vi "SWERVE_DRIVE_SET_SPEED_DEMAND.vi"(8 "Drv Rotation Orentation Dmd":dbl, 9 "Drv Angular Vel Dmd":dbl, 10 "Drv Y Vel Dmd":dbl, 11 "Drv X Vel Dmd":dbl) -> ()   [LabVIEW 2019]
uses:
  SWERVE_DRIVE_GLOBALS.vi
  <vilib>/Rock Robotics/WPI/ThirdParty/JAS_Junk/TrajLib/Trajectory_Library.lvlib
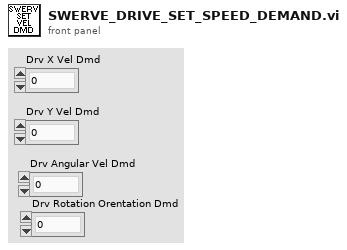
[diagram p1: front panel]
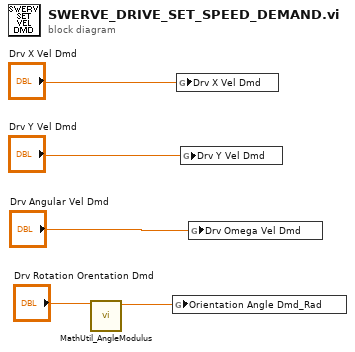
[diagram p0: block diagram]
diagram:
  n1 = call <vilib>:"MathUtil_AngleModulus.vi"("InputAngle"="Drv Rotation Orentation Dmd") -> ("ModulsAngle"=w1:dbl)  [unwired: 10 in]
  n2 = global write "SWERVE_DRIVE_GLOBALS.vi" "Orientation Angle Dmd_Rad"(w1) -> ()
  n3 = global write "SWERVE_DRIVE_GLOBALS.vi" "Drv X Vel Dmd"("Drv X Vel Dmd") -> ()
  n4 = global write "SWERVE_DRIVE_GLOBALS.vi" "Drv Y Vel Dmd"("Drv Y Vel Dmd") -> ()
  n5 = global write "SWERVE_DRIVE_GLOBALS.vi" "Drv Omega Vel Dmd"("Drv Angular Vel Dmd") -> ()
